vi "GetName.vi"() -> ()   [LabVIEW 2014]
panel:
  out "ComputerName":string
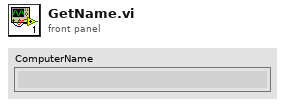
[diagram p1: front panel]
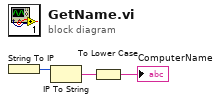
[diagram p0: block diagram]
diagram:
  n1 = String To IP() -> (0:w3:u32)  [unwired: 1 in]
  n2 = IP To String(2:w3) -> (0:w2:string)  [unwired: 1 in]
  n3 = To Lower Case(string=w2) -> (all lower case string=→"ComputerName":string)
